vi "Initialize Transfers.vi"(7 "component name":string, 8 "error in (no error)":errorcluster, 11 "Group Configuration":refnum<class "Group Configuration.lvclass">=refnum) -> (0 "error out":errorcluster, 2 "max buffer size":u64, 3 "transfer parameters":T1[](array[typedef]))   [LabVIEW 2020, in "UDP.lvlib" / "UDP Transceiver.lvclass"]
uses:
  UDP Transceiver.lvclass
  Transfer Parameters.ctl
  Configuration/Tx Transfer/UDP Transfer Tx Configuration.lvclass
  Configuration/Rx Transfer/UDP Transfer Rx Configuration.lvclass
  DSF Core.lvlibp/Classes/Configuration/Core/Transfer/Transfer Configuration.lvclass
  DSF Core.lvlibp/Classes/Configuration/Core/Group/Group Configuration.lvclass
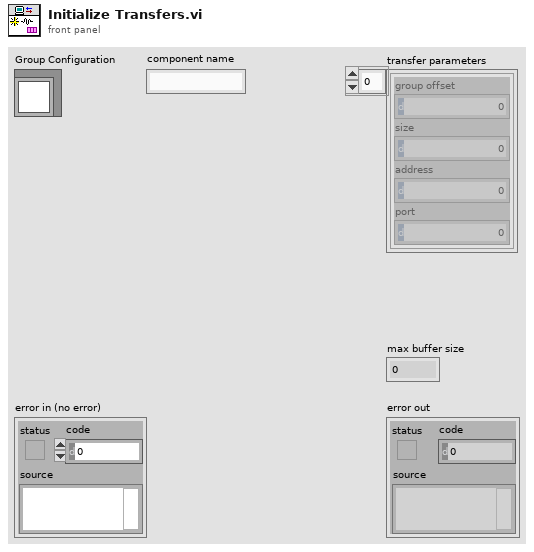
[diagram p1: front panel]
types:
  T1 = typedef "UDP.lvlib/UDP Transceiver.lvclass/Transfer Parameters.ctl" = cluster{"group offset":u64, "size":u64, "address":u32, "port":u16}
  T2 = typedef "DSF Core.lvlibp/Group Configuration.lvclass/Core Group Configuration.ctl" = cluster{"name":string, "direction":T3, "cycle timing":T4, "timeout behavior":T5, "enable conversion":bool}
  T3 = typedef "DSF Core.lvlibp/DSF Direction.ctl" = enum8{"Tx", "Rx"}
  T4 = typedef "DSF Core.lvlibp/DSF Timing Info.ctl" = cluster{"priority":u64, "decimation":u64, "offset":u64}
  T5 = typedef "DSF Core.lvlibp/DSF Timeout Behavior.ctl" = enum8{"Increment Late Count", "Throw Error"}
  T6 = typedef "DSF Core.lvlibp/DSF Settings Info.ctl" = cluster{"component":string, "values":cluster{"key":string, "value":string}[]}
  T7 = typedef "UDP.lvlib/UDP Transfer Tx Configuration.lvclass/Tx Transfer Settings.ctl" = cluster{"address":u32, "port":u16}
  T8 = typedef "UDP.lvlib/UDP Transfer Rx Configuration.lvclass/Rx Transfer Settings.ctl" = cluster{"address":u32, "port":u16}
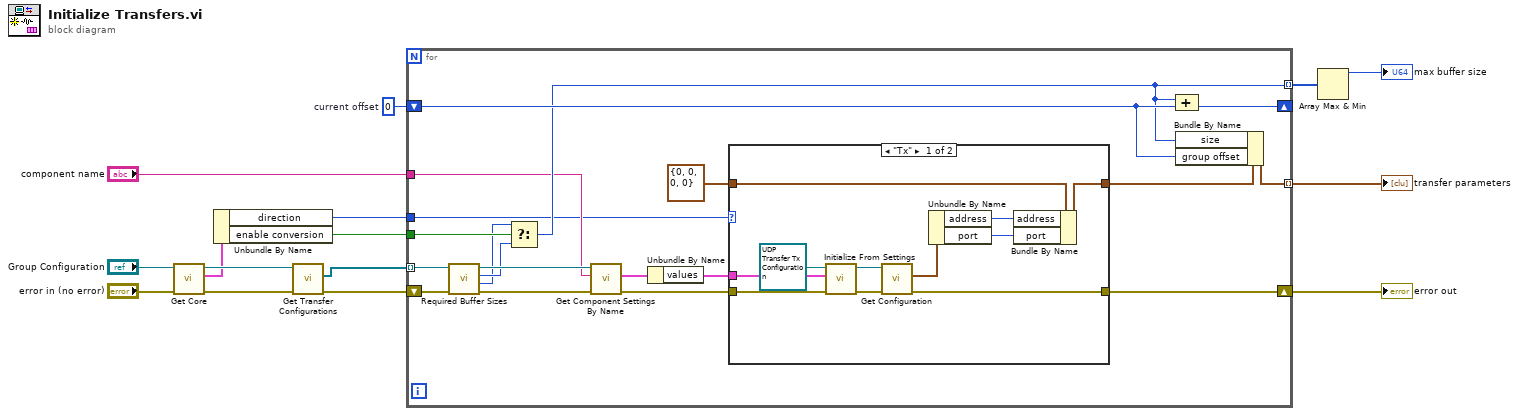
[diagram p0: block diagram]
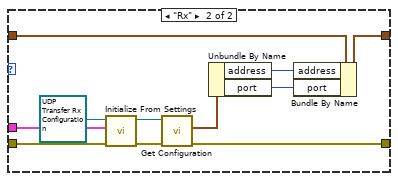
[diagram p2: hidden frame]
diagram:
  w10 = u64 0  # current offset
  n1 = call "Get Core.vi"("error in (no error)"="error in (no error)", "Group Configuration in"="Group Configuration") -> ("error out"=w3:errorcluster, "core"=w7:T2, "Group Configuration out"=w8:refnum<class "Group Configuration.lvclass">)  [unwired: 7 in]
  n2 = Unbundle By Name(w7) -> ("direction"=w11:T3, "enable conversion"=w2:bool)
  n3 = call "Get Transfer Configurations.vi"("error in (no error)"=w3, "Group Configuration in"=w8) -> ("error out"=w4:errorcluster, "Transfer Configurations"=w6:refnum<class "Transfer Configuration.lvclass">[])  [unwired: 7 in, 1 out]
  n4 = for {
    shift-right: [w19] -> w14
    shift-left: w4 -> [w30]
    tunnel: w6 -> [w34] mode=indexing
    tunnel: [w31] -> w15 mode=indexing
    tunnel: [w27] -> w13 mode=indexing
    tunnel: w11 -> [w24]
    shift-right: [w33] -> _
    shift-left: w10 -> [w32]
    tunnel: w2 -> [w26]
    tunnel: "component name" -> [w25]
    n5 = call-dynamic "Required Buffer Sizes.vi"("error in (no error)"=w30, "Transfer Configuration in"=w34) -> ("error out"=w29:errorcluster, "string size"=w16:u64, "engine size"=w17:u64, "Transfer Configuration out"=w28:refnum<class "Transfer Configuration.lvclass">)  [unwired: 6 in]
    n6 = Select(t=w16, s=w26, f=w17) -> (s? t:f=w27:u64)
    n7 = call "Get Component Settings By Name.vi"("error in (no error)"=w29, "component name"=w25, "Runtime Configuration in"=w28) -> ("error out"=w23:errorcluster, "component settings"=w21:T6)  [unwired: 6 in, 1 out]
    n8 = Unbundle By Name(w21) -> ("values"=w20:cluster{"key":string, "value":string}[])
    n9 = case shown="\"Tx\"" w24 {
      tunnel: w23 -> [w45 w51]
      tunnel: T1 {"group offset"=0, "size"=0, "address"=0, "port"=0} ("Transfer Tx") -> [w42 w56]
      tunnel: w20 -> [w44 w46]
      tunnel: [w38 w49] -> w19
      tunnel: [w41 w55] -> w18
      frame "Tx" {
        n10 = call-dynamic "Initialize From Settings.vi"("error in (no error)"=w45, "settings"=w44, "UDP Tx Transfer Configuration in"=refnum<class "UDP Transfer Tx Configuration.lvclass"> refnum) -> ("error out"=w40:errorcluster, "UDP Tx Transfer Configuration out"=w39:refnum<class "UDP Transfer Tx Configuration.lvclass">)  [unwired: 7 in]
        n11 = call "Get Configuration.vi"("error in (no error)"=w40, "UDP Transfer Tx Configuration in"=w39) -> ("error out"=w38:errorcluster, "transfer settings"=w37:T7)  [unwired: 7 in, 1 out]
        n12 = Unbundle By Name(w37) -> ("address"=w36:u32, "port"=w35:u16)
        n13 = Bundle By Name(cluster=w42, "address"=w36, "port"=w35) -> (w41:T1)
      }
      frame "Rx" {
        n14 = call-dynamic "Initialize From Settings.vi"("error in (no error)"=w51, "settings"=w46, "UDP Rx Transfer Configuration in"=refnum<class "UDP Transfer Rx Configuration.lvclass"> refnum) -> ("error out"=w50:errorcluster, "UDP Rx Transfer Configuration out"=w47:refnum<class "UDP Transfer Rx Configuration.lvclass">)  [unwired: 7 in]
        n15 = call "Get Configuration.vi"("error in (no error)"=w50, "UDP Transfer Rx Configuration in"=w47) -> ("error out"=w49:errorcluster, "transfer settings"=w48:T8)  [unwired: 7 in, 1 out]
        n16 = Unbundle By Name(w48) -> ("address"=w54:u32, "port"=w53:u16)
        n17 = Bundle By Name(cluster=w56, "address"=w54, "port"=w53) -> (w55:T1)
      }
    }
    n18 = Compound Arithmetic op=ADD(w27, w32) -> (w33:u64)
    n19 = Bundle By Name(cluster=w18, "size"=w27, "group offset"=w32) -> (w31:T1)
  }
  "error out" <- w14
  "transfer parameters" <- w15
  n20 = Array Max & Min(array=w13) -> (max value=→"max buffer size":u64)  [unwired: 3 out]
